vi "Global.vi"() -> ()   [LabVIEW 2020]
panel:
  in  "Malleable VIs":set{string}(c389)
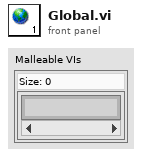
[diagram p1: front panel]
diagram:
